vi "ElmoVelScale.vi"(1 "Elmo eCAT vel":i32) -> (0 "Elmo vel (rev/s)":dbl)   [LabVIEW 2018]
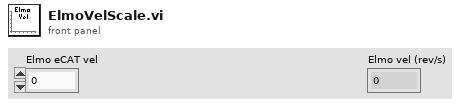
[diagram p1: front panel]
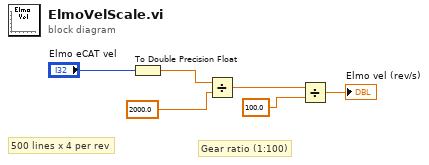
[diagram p0: block diagram]
diagram:
  # "500 lines x 4 per rev"
  # "Gear ratio (1:100)"
  n1 = To Double Precision Float(number="Elmo eCAT vel") -> (double precision float=w6:dbl)
  n2 = Divide(x=w6, y=2000.0) -> (x/y=w4:dbl)
  n3 = Divide(x=w4, y=100.0) -> (x/y=→"Elmo vel (rev/s)":dbl)
